vi "Unknown.vi"   [LabVIEW 2014]
types:
  T1 = typedef "WPI_CompressorDevRef.ctl" = cluster{"DevStatus":errorcluster, "Pneumatics Control Module":u8}
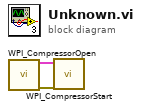
[diagram p0: block diagram]
diagram:
  n1 = call <vilib>:"WPI_CompressorOpen.vi"() -> ("CompressorDevRef"=w1:T1, "error out"=w2:errorcluster)  [unwired: 14 in]
  n2 = call <vilib>:"WPI_CompressorStart.vi"("error in (no error)"=w2, "CompressorDevRef"=w1) -> ()  [unwired: 8 in, 2 out]
